vi "Read ILC Serial Settings.vi"(8 "error in (no error)":errorcluster, 11 "Boot Loader in":refnum<class "Boot Loader.lvclass">) -> (0 "error out":errorcluster, 2 "Serial Settings":T1={"Baud Rate"=9600, "Data Bits"=8, "Parity"=enum."None", "Flow Control"=0, "Stop Bits"=10, "Timeout (ms)"=10000, "Byte Count"=200, "Enable Termination Character"=FALSE, "Termination Char"=200} {"Termination Char" format="%x"; "Stop Bits" items=["1.0"=10, "1.5"=15, "2.0"=20]; "Flow Control" items=["None", "XON/XOFF", "RTS/CTS", "XON/XOFF & RTS/CTS", "DTR/DSR", "XON/XOFF & DTR/DSR"]; "Data Bits" min=5 max=8 step=1}, 3 "Boot Loader out":refnum<class "Boot Loader.lvclass">)   [LabVIEW 2016, in "Boot Loader.lvclass"]
uses:
  Boot Loader.lvclass
  Typedefs/SerialSettings.ctl
  Settings/Settings.lvclass
  Typedefs/HPMT_Typedefs.lvlib
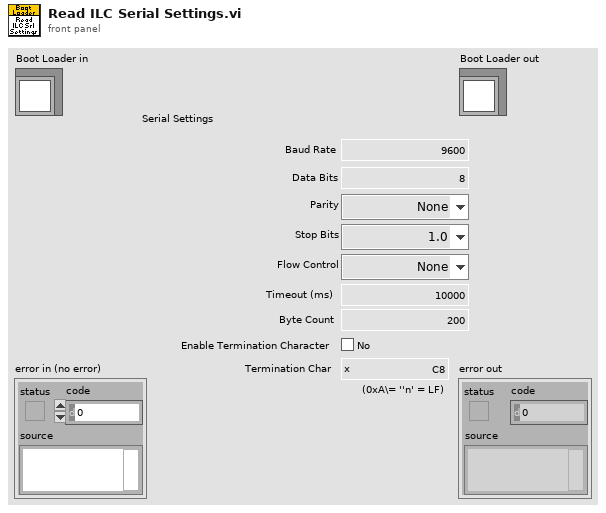
[diagram p1: front panel]
types:
  T1 = typedef "HPMT_Typedefs.lvlib/SerialSettings.ctl" = cluster{"Baud Rate":u32, "Data Bits":u16, "Parity":enum16{"None", "Odd", "Even", "Mark", "Space"}, "Flow Control":u16, "Stop Bits":u16, "Timeout (ms)":u32, "Byte Count":u32, "Enable Termination Character":bool, "Termination Char":u8}
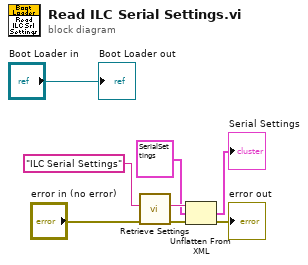
[diagram p0: block diagram]
diagram:
  n1 = call "Retrieve Settings.vi"("error in (no error)"="error in (no error)", "configName"="ILC Serial Settings") -> ("error out"=w4:errorcluster, "xmlConfig"=w7:string)  [unwired: 7 in, 1 out]
  n2 = Unflatten From XML(xml string=w7, type=T1 {"Baud Rate"=9600, "Data Bits"=8, "Parity"=enum."None", "Flow Control"=0, "Stop Bits"=10, "Timeout (ms)"=10000, "Byte Count"=200, "Enable Termination Character"=FALSE, "Termination Char"=200} ("Serial Settings"), error in (no error)=w4) -> (value=→"Serial Settings":T1, error out=→"error out":errorcluster)
  "Boot Loader out" <- "Boot Loader in"
